vi "Main_ultra.vi"() -> ()   [LabVIEW 2020]
uses:
  <vilib>/Platform/TimedLoop/XDataNode/timing_clust.ctl
  <vilib>/Platform/TimedLoop/XDataNode/nitl_modes.ctl
  <vilib>/Platform/TimedLoop/XDataNode/wakeup.ctl
  <vilib>/Platform/TimedLoop/XDataNode/loadnilvce.vi
  <vilib>/imath/engines/lvmath2/RunTimeEngine/Managers/WorkSpace/UID Generator.vi
  <vilib>/imath/engines/lvmath2/RunTimeEngine/RunTimeType/NIMS_RunTimeType_From StrictType (excl LVString).vi
  <instcachedir>/0/NIMS_RunTimeType_From StrictType (excl LVString)_283B1B2000484AAA8744D21CE97EA49F.lvgen/NIMS_RunTimeType_From StrictType (excl LVString)_283B1B2000484AAA8744D21CE97EA49F_000.vi
  <vilib>/imath/engines/lvmath2/RunTimeEngine/LocalVariableDefStatement/MC_LocalVariableDefStatement_Display.vi
  <vilib>/imath/engines/lvmath2/RunTimeEngine/BuiltInFunctions/round/NIMS_round(DBL-S).vi
  <vilib>/imath/engines/lvmath2/RunTimeEngine/RunTimeType/NIMS_RunTimeType_Set Source Original Bool.vi
  <vilib>/imath/engines/lvmath2/RunTimeEngine/Managers/SymbolTable/Clear UID.vi
  <vilib>/imath/engines/lvmath2/RunTimeEngine/NodeEndStatement/NIMS_NodeEndStatement_Output.vi
  <instcachedir>/0/NIMS_NodeEndStatement_Output_53EC0D466D134D7ABD903AC30B43404B.lvgen/NIMS_NodeEndStatement_Output_53EC0D466D134D7ABD903AC30B43404B_001.vi
  <instcachedir>/0/NIMS_NodeEndStatement_Output_53EC0D466D134D7ABD903AC30B43404B.lvgen/NIMS_NodeEndStatement_Output_53EC0D466D134D7ABD903AC30B43404B_010.vi
  <vilib>/imath/engines/lvmath2/RunTimeEngine/ErrorHandling/NIMS_Finalize Error.vi
  Global 2.vi
  <instcachedir>/0/NIMS_NodeEndStatement_Output_53EC0D466D134D7ABD903AC30B43404B.lvgen/NIMS_NodeEndStatement_Output_53EC0D466D134D7ABD903AC30B43404B_005.vi
  <vilib>/imath/engines/lvmath2/RunTimeEngine/CommandStatement/MC_CommandStatement_break.vi
  <vilib>/imath/engines/lvmath2/RunTimeEngine/IndexReplace/NIMS M(S,S)=S.vi
  <instcachedir>/0/NIMS M(S,S)=S_FBAB070788A64735BCFA47F7F92815DB.lvgen/NIMS M(S,S)=S_FBAB070788A64735BCFA47F7F92815DB_000.vi
  <vilib>/imathl/engines/lvmath/Functions/Error Handling/Create Error.vi
  <instcachedir>/0/NIMS M(S,S)=S_FBAB070788A64735BCFA47F7F92815DB.lvgen/NIMS M(S,S)=S_FBAB070788A64735BCFA47F7F92815DB_002.vi
  <vilib>/imath/engines/lvmath2/RunTimeEngine/CommandStatement/NIMS_CommandStatement_MaskErr.vi
  <vilib>/imath/engines/lvmath2/RunTimeEngine/ArithmeticOperatorToken/NIMS_ArithmeticOperator_multmx-internal.vi
  <instcachedir>/0/NIMS_ArithmeticOperator_multmx-internal_B44B9A6937C8407A9A8862E3F2935EB3.lvgen/NIMS_ArithmeticOperator_multmx-internal_B44B9A6937C8407A9A8862E3F2935EB3_004.vi
  <vilib>/imath/engines/lvmath2/RunTimeEngine/BuiltInFunctions/length/NIMS_length(GM).vi
  <instcachedir>/0/NIMS_length(GM)_47CEC356FCE0482D9BA47DC61C99F2C7.lvgen/NIMS_length(GM)_47CEC356FCE0482D9BA47DC61C99F2C7_000.vi
  <vilib>/imath/engines/lvmath2/RunTimeEngine/RangeToken/NIMS_Range_R2 - Integer.vi
  <instcachedir>/0/NIMS_Range_R2 - Integer_FFC1A4B1B9F04947ABCB56F009996D55.lvgen/NIMS_Range_R2 - Integer_FFC1A4B1B9F04947ABCB56F009996D55_000.vi
  <vilib>/imath/engines/lvmath2/RunTimeEngine/IndexRead/NIMS M(S).vi
  <instcachedir>/0/NIMS M(S)_B826C018497E4940AE96BD27B540B6FB.lvgen/NIMS M(S)_B826C018497E4940AE96BD27B540B6FB_000.vi
  <instcachedir>/0/NIMS M(S)_B826C018497E4940AE96BD27B540B6FB.lvgen/NIMS M(S)_B826C018497E4940AE96BD27B540B6FB_005.vi
  <vilib>/imath/engines/lvmath2/RunTimeEngine/ArithmeticOperatorToken/NIMS_ArithmeticOperator_multmx(M,CV)-internal.vi
  <instcachedir>/0/NIMS_ArithmeticOperator_multmx(M,CV)-internal_19A14CC5BE0A4D31BE1E94A2E998D8C3.lvgen/NIMS_ArithmeticOperator_multmx(M,CV)-internal_19A14CC5BE0A4D31BE1E94A2E998D8C3_001.vi
  <vilib>/imath/engines/lvmath2/RunTimeEngine/IndexReplace/NIMS M($,S)=V.vi
  <instcachedir>/0/NIMS M($,S)=V_85A28EB895514E96A13A10261726EE3A.lvgen/NIMS M($,S)=V_85A28EB895514E96A13A10261726EE3A_001.vi
  <vilib>/imath/engines/lvmath2/RunTimeEngine/ErrorHandling/NIMS_Create Error From Enums.vi
  <vilib>/imath/engines/lvmath2/RunTimeEngine/RowToken/NIMS_RowToken_M_M.vi
  <instcachedir>/0/NIMS_RowToken_M_M_23B851CD98934479877138710C79658F.lvgen/NIMS_RowToken_M_M_23B851CD98934479877138710C79658F_004.vi
  <instcachedir>/0/NIMS_NodeEndStatement_Output_53EC0D466D134D7ABD903AC30B43404B.lvgen/NIMS_NodeEndStatement_Output_53EC0D466D134D7ABD903AC30B43404B_002.vi
  <vilib>/imath/engines/lvmath2/RunTimeEngine/BuiltInFunctions/size/NIMS_[I32,I32]=size(GM).vi
  <instcachedir>/0/NIMS_[I32,I32]=size(GM)_B0A6EC1255BB4C8AB801FE6F734128D9.lvgen/NIMS_[I32,I32]=size(GM)_B0A6EC1255BB4C8AB801FE6F734128D9_000.vi
  <vilib>/imath/engines/lvmath2/RunTimeEngine/BuiltInFunctions/zeros/NIMS_V=zeros(I32,I32).vi
  <vilib>/imath/engines/lvmath2/RunTimeEngine/IndexRead/NIMS M($,S).vi
  <instcachedir>/0/NIMS M($,S)_3E5749BBB62E49528D4765A77F1F6D98.lvgen/NIMS M($,S)_3E5749BBB62E49528D4765A77F1F6D98_000.vi
  <vilib>/imath/engines/lvmath2/RunTimeEngine/ArithmeticOperatorToken/NIMS_ArithmeticOperator_plus.vi
  <instcachedir>/0/NIMS_ArithmeticOperator_plus_54468E2FAC2848C4BF0D457641184E60.lvgen/NIMS_ArithmeticOperator_plus_54468E2FAC2848C4BF0D457641184E60_004.vi
  <vilib>/imath/engines/lvmath2/RunTimeEngine/RowToken/NIMS_RowToken_CV_CV.vi
  <instcachedir>/0/NIMS_RowToken_CV_CV_E2834F2F68C5494A92C49C498959A73E.lvgen/NIMS_RowToken_CV_CV_E2834F2F68C5494A92C49C498959A73E_000.vi
  <vilib>/imath/engines/lvmath2/RunTimeEngine/RowToken/NIMS_RowToken_M_CV.vi
  <instcachedir>/0/NIMS_RowToken_M_CV_79C297319A314039B767729C6880A213.lvgen/NIMS_RowToken_M_CV_79C297319A314039B767729C6880A213_000.vi
  <vilib>/imath/engines/lvmath2/RunTimeEngine/IndexRead/NIMS M(S,$).vi
  <instcachedir>/0/NIMS M(S,$)_F24F360562DE41D8BE234322A2E15C65.lvgen/NIMS M(S,$)_F24F360562DE41D8BE234322A2E15C65_000.vi
  <vilib>/imath/engines/lvmath2/RunTimeEngine/IndexReplace/NIMS M(S)=S.vi
  <instcachedir>/0/NIMS M(S)=S_033E230F5F1E47BAA81748F03F1A64B6.lvgen/NIMS M(S)=S_033E230F5F1E47BAA81748F03F1A64B6_001.vi
  <vilib>/imath/engines/lvmath2/RunTimeEngine/NodeEndStatement/NIMS_NodeEndStatement_Get Vector.vi
  <instcachedir>/0/NIMS_NodeEndStatement_Get Vector_F9EEA26507564AFBA1E30D500A99934B.lvgen/NIMS_NodeEndStatement_Get Vector_F9EEA26507564AFBA1E30D500A99934B_001.vi
  <vilib>/imath/engines/lvmath/Functions/Error Handling/MergeErrorsWrapper.vi
  <vilib>/imath/engines/lvmath2/RunTimeEngine/IndexRead/NIMS V(S).vi
  <instcachedir>/0/NIMS V(S)_0488751826AF41519A22953C041130DC.lvgen/NIMS V(S)_0488751826AF41519A22953C041130DC_000.vi
  <vilib>/imath/engines/lvmath2/RunTimeEngine/BuiltInFunctions/norm/NIMS_norm(GV,DBL).vi
  <instcachedir>/0/NIMS_norm(GV,DBL)_118B4CCB667A4D7498CD7C123070720C.lvgen/NIMS_norm(GV,DBL)_118B4CCB667A4D7498CD7C123070720C_000.vi
  <vilib>/imath/engines/lvmath2/RunTimeEngine/BuiltInFunctions/cos/NIMS_cos(C).vi
  <instcachedir>/0/NIMS_cos(C)_9DC0D0878EF24EB8B280F2BED1FF8FCD.lvgen/NIMS_cos(C)_9DC0D0878EF24EB8B280F2BED1FF8FCD_001.vi
  <vilib>/imath/engines/lvmath2/RunTimeEngine/BuiltInFunctions/acos/NIMS_acos(C).vi
  <instcachedir>/0/NIMS_acos(C)_5BB0E87CCFB0408A9DC8B350AC83525E.lvgen/NIMS_acos(C)_5BB0E87CCFB0408A9DC8B350AC83525E_001.vi
  <instcachedir>/0/NIMS_RunTimeType_From StrictType (excl LVString)_283B1B2000484AAA8744D21CE97EA49F.lvgen/NIMS_RunTimeType_From StrictType (excl LVString)_283B1B2000484AAA8744D21CE97EA49F_009.vi
  <vilib>/imath/engines/lvmath2/RunTimeEngine/BuiltInFunctions/abs/NIMS_abs(signed).vi
  <instcachedir>/0/NIMS_abs(signed)_C4FCB8E6058B49B797C7C8D53CA5F6EC.lvgen/NIMS_abs(signed)_C4FCB8E6058B49B797C7C8D53CA5F6EC_002.vi
  <instcachedir>/0/NIMS_NodeEndStatement_Output_53EC0D466D134D7ABD903AC30B43404B.lvgen/NIMS_NodeEndStatement_Output_53EC0D466D134D7ABD903AC30B43404B_009.vi
  <vilib>/platform/TimedLoop/XDataNode/XDataNode.xnode
  <vilib>/Platform/TimedLoop/XDataNode/XDNodeRunTimeDep.lvlib
  <vilib>/imath/engines/lvmath2/RunTimeEngine/Managers/SymbolTable/NIMS_WorkSpace.lvlib
panel:
  out "Temperature":dbl=43.13496907791888
  out "VoltageSaturating":bool
  out "Power":bool
  in  "Power On/Off":bool
  in  "BMagnitude [T]":dbl=0.02
  out "RotationPerSecond[Hz]":dbl=-94.24777499999999
  in  "RotationsPerSecond [Hz]":dbl=-20.0
  out "AngleX":cluster{dbl, dbl}(graph)
  in  "Max Orientation\n change rate [rad/s]":dbl=30.0
  in  "Force Vertical":bool
  in  "Scalar":dbl=0.004
  out "F":dbl=-596.1678650885794
  in  "Reset Integral":bool
  in  "Kp":dbl=40.0
  in  "Ki":dbl=0.001
  in  "Kd":dbl
  out "XY View":T1(graph)=[{"XCircleBot"=[0.03623369648886077, 0.03598886161264151, 0.035314301100597044, 0.034375170892196175, 0.03340140281576648, 0.0326314092577669, 0.03225371149565987, 0.032360783114279174, 0.03292640924713354, 0.03381210488999921, 0.034801020859787216, 0.03565103603744329, 0.0361540370621615], "YCircleBot"=[0.0012174224381933385, 0.0021762735154017446, 0.002900364407809132, 0.0032124124114014476, 0.0030360172918447023, 0.002414366726401252, 0.001499662454313073, 0.0005158559828140988, -0.00029618255242251797, -0.0007376377971368554, -0.0007004261111329384, -0.00019365821294744547, 0.0006585914417954867]}, {"XCircleBot"=[0.0, -0.00199, -0.004019999999999999, -0.0061200000000000004, -0.00816, -0.01026, -0.01234, -0.01435, -0.01622, -0.01804, -0.019920000000000004, -0.02168, -0.02325, -0.02478, -0.02623, -0.02775, -0.02913, -0.030440000000000002, -0.03164, -0.032729999999999995, -0.0337, -0.03456, -0.03524, -0.035840000000000004, -0.03629, -0.03668, -0.03701, -0.03726, -0.037469999999999996, -0.037590000000000005, -0.037630000000000004, -0.03762, -0.03754, -0.037450000000000004, -0.03697, -0.03612, -0.03502, -0.03358, -0.03181, -0.029840000000000002, -0.027800000000000002, -0.0257, -0.023629999999999998, -0.02158, -0.01957, -0.01754, -0.01551, -0.01343, -0.01131, -0.00925, -0.00714, -0.00525, -0.0035499999999999998, -0.00213, -0.0010500000000000002, -0.00041, -3e-05, 0.00047, 0.00132, 0.00252, 0.00405, 0.0057599999999999995, 0.00772, 0.00973, 0.01173, 0.013960000000000002, 0.0162, 0.01825, 0.02047, 0.02266, 0.02475, 0.026760000000000003, 0.028820000000000002, 0.03086, 0.03277, 0.03442, 0.0357, 0.0366, 0.037200000000000004, 0.037520000000000005, 0.03764, 0.037649999999999996, 0.037590000000000005, 0.037520000000000005, 0.037469999999999996, 0.03746, 0.037469999999999996, 0.03749, 0.0375, 0.03751, 0.03751, 0.03751, 0.03751, 0.03751, 0.0375, 0.0375, 0.0375, 0.0375, 0.0375, 0.0375, 0.0375, 0.0375, 0.0375, 0.0375, 0.0375, 0.0375, 0.0375, 0.0375, 0.0375, 0.0375, 0.0375, 0.0375, 0.0375, 0.0375, 0.0375, 0.0375, 0.0375, 0.03751, 0.03751, 0.0375, 0.03748, 0.037469999999999996, 0.037469999999999996, 0.03746, 0.03746, 0.037469999999999996, 0.03749, 0.03753, 0.03758, 0.037630000000000004, 0.03764, 0.0375, 0.03712, 0.03649, 0.0356, 0.034350000000000006, 0.03275, 0.0308, 0.02878, 0.02666, 0.02456, 0.02236, 0.02014, 0.01796, 0.01591, 0.01368, 0.01167, 0.009519999999999999, 0.00723, 0.00479, 0.0027300000000000002, 0.0005600000000000001, 0.0], "YCircleBot"=[-0.0375, -0.03775, -0.03756, -0.03716, -0.03663, -0.03598, -0.035250000000000004, -0.03448, -0.0337, -0.03286, -0.03188, -0.03074, -0.02947, -0.028059999999999998, -0.02664, -0.025050000000000003, -0.0235, -0.02189, -0.020239999999999998, -0.01853, -0.01672, -0.01477, -0.01286, -0.01078, -0.00881, -0.0067800000000000004, -0.004730000000000001, -0.00269, -0.00048, 0.00161, 0.00372, 0.0057599999999999995, 0.00785, 0.009869999999999999, 0.01182, 0.01365, 0.0154, 0.01682, 0.01777, 0.0183, 0.018600000000000002, 0.01875, 0.01881, 0.01881, 0.01877, 0.01871, 0.0187, 0.01878, 0.01886, 0.018760000000000002, 0.01833, 0.01753, 0.016370000000000003, 0.01494, 0.01318, 0.01114, 0.00903, 0.0069500000000000004, 0.00512, 0.0034700000000000004, 0.0020099999999999996, 0.00092, 0.0003, 8e-05, 1e-05, -2e-05, -3e-05, -3e-05, -2e-05, -1e-05, 0.0, 0.0, 0.0, 0.0, 0.0, 0.0, 0.0, 0.0, 0.0, 0.0, 0.0, 0.0, 0.0, 0.0, 1e-05, 1e-05, 2e-05, 1e-05, 0.0, -2e-05, -5e-05, -8.999999999999999e-05, -0.00016, -0.00025, -0.00039000000000000005, -0.00063, -0.0011899999999999999, -0.00279, -0.00452, -0.00628, -0.008150000000000001, -0.01018, -0.01219, -0.01428, -0.016329999999999997, -0.01837, -0.020489999999999998, -0.022600000000000002, -0.02475, -0.02677, -0.02884, -0.03083, -0.03264, -0.03432, -0.03574, -0.03672, -0.0373, -0.03749, -0.0375, -0.0375, -0.0375, -0.0375, -0.0375, -0.0375, -0.0375, -0.0375, -0.0375, -0.0375, -0.0375, -0.0375, -0.0375, -0.0375, -0.0375, -0.0375, -0.0375, -0.0375, -0.0375, -0.0375, -0.0375, -0.0375, -0.0375, -0.0375, -0.0375, -0.0375, -0.0375, -0.0375, -0.0375, -0.0375, -0.0375, -0.0375, -0.0375, -0.0375, -0.0375]}, {"XCircleBot"=[0.02876, 0.028515165123780748, 0.02784060461173628, 0.02690147440333541, 0.025927706326905716, 0.025157712768906135, 0.024780015006799112, 0.02488708662541841, 0.02545271275827278, 0.026338408401138443, 0.027327324370926456, 0.028177339548582522, 0.028680340573300735], "YCircleBot"=[0.0, 0.000958851077208406, 0.0016829419696157931, 0.001994989973208109, 0.0018185948536513636, 0.0011969442882079132, 0.0002822400161197344, -0.0007015664553792397, -0.0015136049906158565, -0.001955060235330194, -0.001917848549326277, -0.001411080651140784, -0.0005588309963978518]}, {"XCircleBot"=[0.034233696488860765, 0.035873148282011894], "YCircleBot"=[0.0012174224381933385, 0.0004059623274943767]}]
  out "XZ View":T1(graph)=[{"XCircleBot"=[0.03623369648886077, 0.03598886161264151, 0.035314301100597044, 0.034375170892196175, 0.03340140281576648, 0.0326314092577669, 0.03225371149565987, 0.032360783114279174, 0.03292640924713354, 0.03381210488999921, 0.034801020859787216, 0.03565103603744329, 0.0361540370621615], "YCircleBot"=[-0.07416133745930864, -0.07320248638210024, -0.07247839548969284, -0.07216634748610053, -0.07234274260565728, -0.07296439317110073, -0.0738790974431889, -0.07486290391468788, -0.0756749424499245, -0.07611639769463883, -0.07607918600863492, -0.07557241811044943, -0.07472016845570649]}, {"XCircleBot"=[0.0, -0.00199, -0.004019999999999999, -0.0061200000000000004, -0.00816, -0.01026, -0.01234, -0.01435, -0.01622, -0.01804, -0.019920000000000004, -0.02168, -0.02325, -0.02478, -0.02623, -0.02775, -0.02913, -0.030440000000000002, -0.03164, -0.032729999999999995, -0.0337, -0.03456, -0.03524, -0.035840000000000004, -0.03629, -0.03668, -0.03701, -0.03726, -0.037469999999999996, -0.037590000000000005, -0.037630000000000004, -0.03762, -0.03754, -0.037450000000000004, -0.03697, -0.03612, -0.03502, -0.03358, -0.03181, -0.029840000000000002, -0.027800000000000002, -0.0257, -0.023629999999999998, -0.02158, -0.01957, -0.01754, -0.01551, -0.01343, -0.01131, -0.00925, -0.00714, -0.00525, -0.0035499999999999998, -0.00213, -0.0010500000000000002, -0.00041, -3e-05, 0.00047, 0.00132, 0.00252, 0.00405, 0.0057599999999999995, 0.00772, 0.00973, 0.01173, 0.013960000000000002, 0.0162, 0.01825, 0.02047, 0.02266, 0.02475, 0.026760000000000003, 0.028820000000000002, 0.03086, 0.03277, 0.03442, 0.0357, 0.0366, 0.037200000000000004, 0.037520000000000005, 0.03764, 0.037649999999999996, 0.037590000000000005, 0.037520000000000005, 0.037469999999999996, 0.03746, 0.037469999999999996, 0.03749, 0.0375, 0.03751, 0.03751, 0.03751, 0.03751, 0.03751, 0.0375, 0.0375, 0.0375, 0.0375, 0.0375, 0.0375, 0.0375, 0.0375, 0.0375, 0.0375, 0.0375, 0.0375, 0.0375, 0.0375, 0.0375, 0.0375, 0.0375, 0.0375, 0.0375, 0.0375, 0.0375, 0.0375, 0.0375, 0.03751, 0.03751, 0.0375, 0.03748, 0.037469999999999996, 0.037469999999999996, 0.03746, 0.03746, 0.037469999999999996, 0.03749, 0.03753, 0.03758, 0.037630000000000004, 0.03764, 0.0375, 0.03712, 0.03649, 0.0356, 0.034350000000000006, 0.03275, 0.0308, 0.02878, 0.02666, 0.02456, 0.02236, 0.02014, 0.01796, 0.01591, 0.01368, 0.01167, 0.009519999999999999, 0.00723, 0.00479, 0.0027300000000000002, 0.0005600000000000001, 0.0], "YCircleBot"=[0.0, 0.0, 0.0, 0.0, 0.0, 0.0, 0.0, 0.0, 0.0, 0.0, 0.0, 0.0, 0.0, 0.0, 0.0, 0.0, 0.0, 0.0, 0.0, 0.0, 0.0, 0.0, 0.0, 0.0, 0.0, 0.0, 0.0, 0.0, 0.0, 0.0, 0.0, 0.0, 0.0, 0.0, 0.0, 0.0, 0.0, 0.0, 0.0, 0.0, 0.0, 0.0, 0.0, 0.0, 0.0, 0.0, 0.0, 0.0, 0.0, 0.0, 0.0, 0.0, 0.0, 0.0, 0.0, 0.0, 0.0, 0.0, 0.0, 0.0, 0.0, 0.0, 0.0, 0.0, 0.0, 0.0, 1e-05, 1e-05, 1e-05, 1e-05, -1e-05, -4e-05, 0.00017, 0.00063, 0.00143, 0.0027, 0.00435, 0.00619, 0.00816, 0.01016, 0.012230000000000001, 0.01425, 0.01629, 0.0183, 0.02036, 0.0224, 0.02442, 0.02655, 0.028800000000000003, 0.03081, 0.032979999999999995, 0.03522, 0.03744, 0.039549999999999995, 0.0417, 0.04382, 0.045770000000000005, 0.047, 0.048049999999999995, 0.04915, 0.049890000000000004, 0.05004, 0.04999, 0.04997, 0.04998, 0.04999, 0.05001, 0.05002, 0.05002, 0.05001, 0.04995, 0.049479999999999996, 0.04846, 0.047200000000000006, 0.045700000000000005, 0.043930000000000004, 0.042, 0.039939999999999996, 0.037880000000000004, 0.03587, 0.03356, 0.03125, 0.02913, 0.026949999999999998, 0.02477, 0.02266, 0.02036, 0.01833, 0.016100000000000003, 0.014060000000000001, 0.012029999999999999, 0.01, 0.00795, 0.006030000000000001, 0.00421, 0.0025499999999999997, 0.00132, 0.00055, 0.00017999999999999998, 3e-05, -2e-05, -2e-05, 1e-05, 4e-05, 7.000000000000001e-05, 8.999999999999999e-05, 0.0001, 0.00011, 0.0001, 8e-05, 5e-05, 1e-05, 0.0]}, {"XCircleBot"=[0.02876, 0.028515165123780748, 0.02784060461173628, 0.02690147440333541, 0.025927706326905716, 0.025157712768906135, 0.024780015006799112, 0.02488708662541841, 0.02545271275827278, 0.026338408401138443, 0.027327324370926456, 0.028177339548582522, 0.028680340573300735], "YCircleBot"=[-4e-05, 0.000918851077208406, 0.001642941969615793, 0.001954989973208109, 0.0017785948536513635, 0.001156944288207913, 0.0002422400161197344, -0.0007415664553792397, -0.0015536049906158566, -0.001995060235330194, -0.001957848549326277, -0.001451080651140784, -0.0005988309963978518]}, {"XCircleBot"=[0.034233696488860765, 0.035873148282011894], "YCircleBot"=[-0.07416133745930864, -0.024194811361262974]}]
  in  "Ahead":dbl=1.0 format="%#_13g"
  out "Error":dbl(graph)=0.07450711995076267
  out "error":cdb=0.07450711995076267+0.0i
  in  "Radio Buttons":enum32{"Stadium", "Circle"}(radio)
  in  "Zscale":dbl=0.95
  in  "YScale":dbl=0.9
  in  "XScale":dbl=0.95
  in  "Zoffset":dbl=-0.073
  in  "Yoffset":dbl=-0.076
  in  "Xoffset":dbl=0.07
  in  "Traj_Rotate":bool
  in  "stop":bool
  out "Loop Duration [ms]":u32
  in  "Settings 4":T2={"Objects"=1, "Threshold"=95, "Reject Border"=FALSE, "Fill Holes"=FALSE, "Min Object Size"=TRUE, "Min Size"=25, "Max Object Size"=TRUE, "Max Size"=25000, "Show Search Area"=TRUE, "Show Center"=TRUE, "Show Bounding Box"=TRUE} {"Objects" items=["Bright Objects", "Dark Objects"]; "Threshold" min=1 max=999999999 step=1; "Max Size" min=1 max=999999999 step=1; "Min Size" min=1 max=999999999 step=1}
  out "Image 4":T3(plugin-control)
  in  "Settings 3":T2={"Objects"=1, "Threshold"=1, "Reject Border"=FALSE, "Fill Holes"=FALSE, "Min Object Size"=TRUE, "Min Size"=25, "Max Object Size"=TRUE, "Max Size"=25000, "Show Search Area"=FALSE, "Show Center"=TRUE, "Show Bounding Box"=TRUE} {"Objects" items=["Bright Objects", "Dark Objects"]; "Threshold" min=1 max=999999999 step=1; "Max Size" min=1 max=999999999 step=1; "Min Size" min=1 max=999999999 step=1}
  out "Image 3":T3(plugin-control)
  in  "Vision compensation":bool=TRUE
  out "Vision compensation active":bool=TRUE
  out "coordinates":cluster{dbl, dbl, dbl}(graph)={0.0027, -0.0171, 0.0805}
  out "camera rate":u32=11
  out "X":dbl=0.0027
  out "Y":dbl=-0.0171
  out "Z":dbl=0.0805
  out "Error_detection":bool
  out "Detection_Error":cdb
  in  "Search Rect (entire image)":T4={"Left"=224, "Top"=459, "Right"=496, "Bottom"=249, "Rotation"=0.0} {"Rotation" format="%.2f"; "Left" scale=0.0..1024.0; "Right" scale=0.0..1024.0}
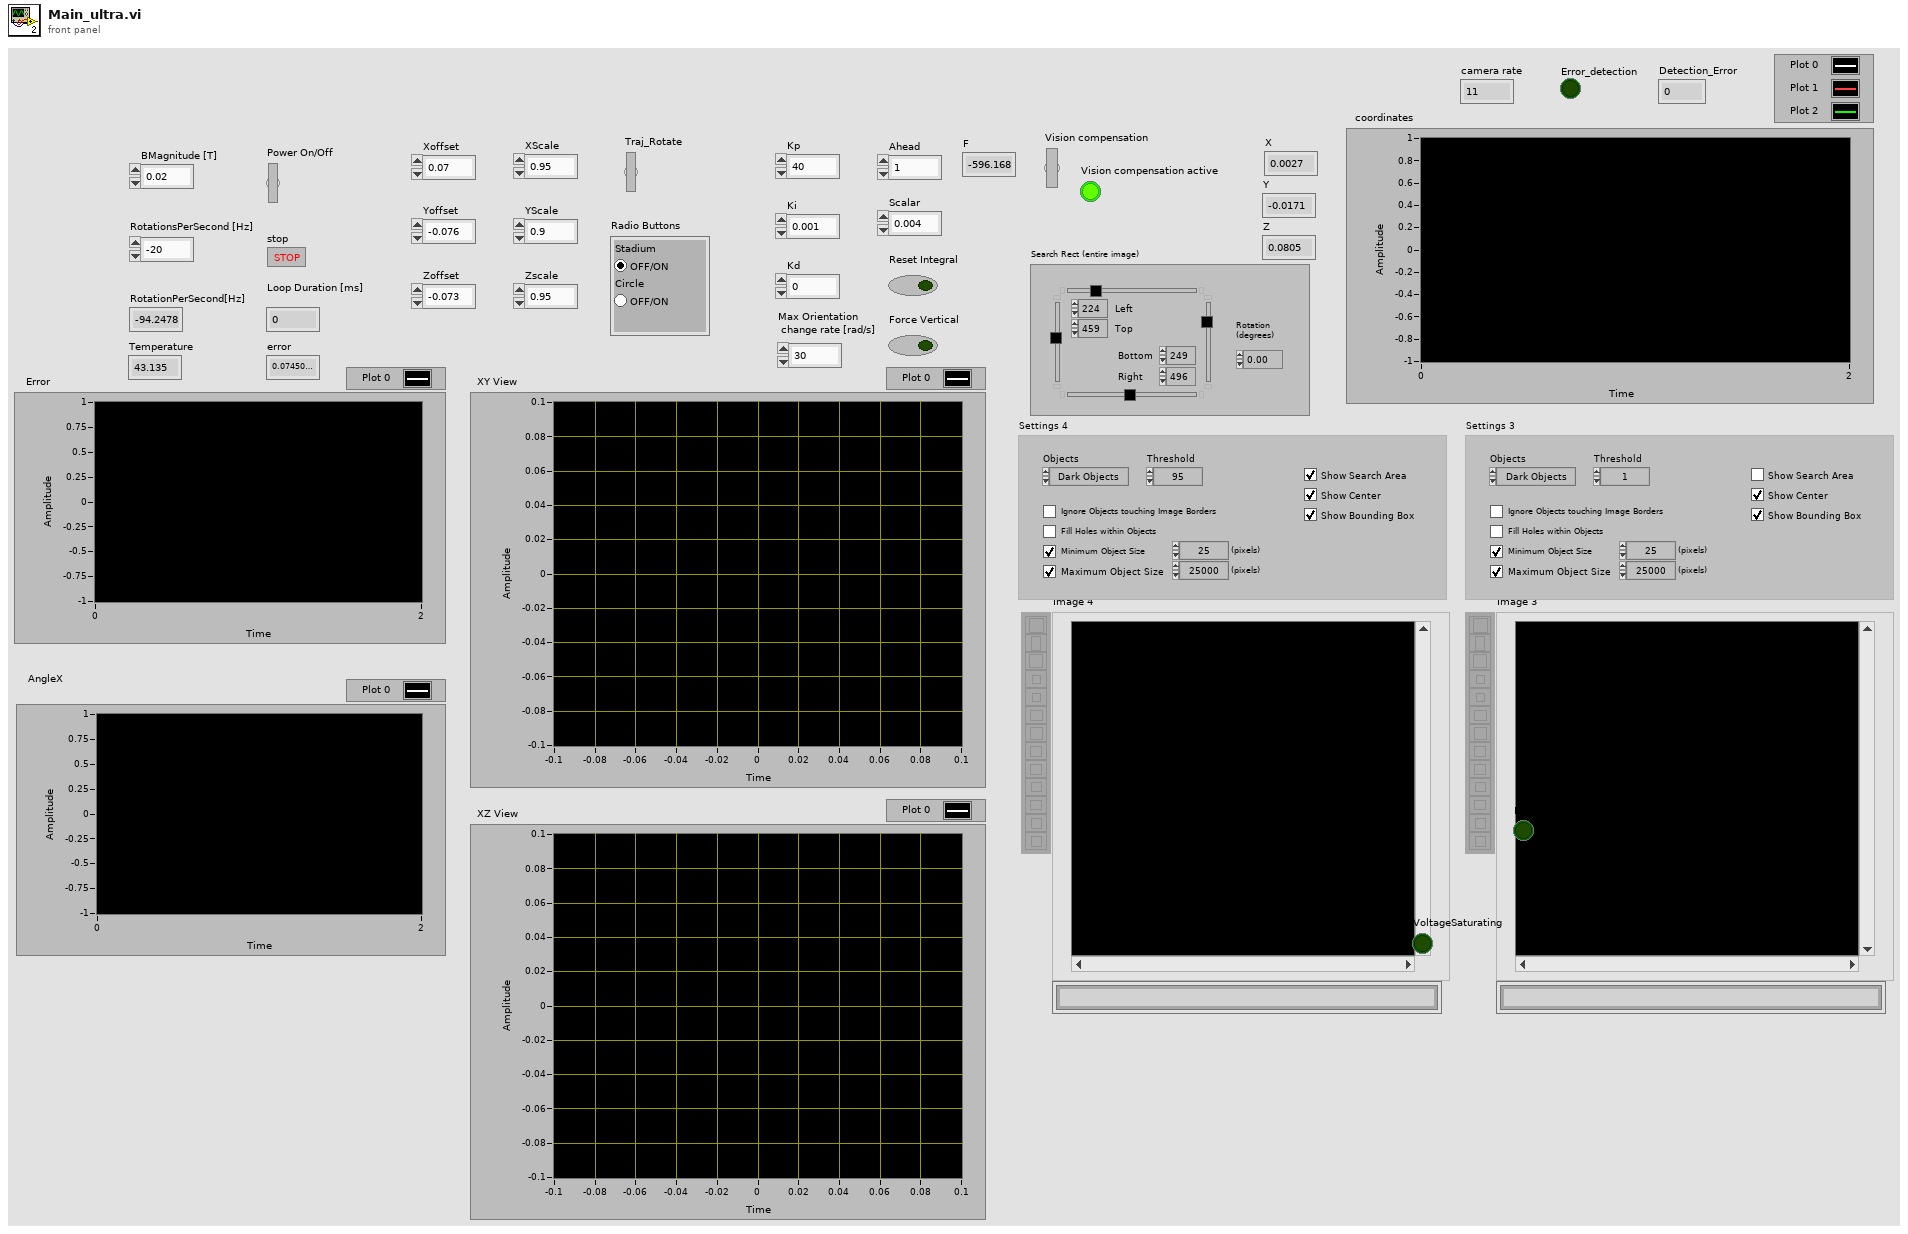
[diagram p1: front panel]
types:
  T1 = cluster{"XCircleBot":dbl[], "YCircleBot":dbl[]}[]
  T2 = cluster{"Objects":u16, "Threshold":i32, "Reject Border":bool, "Fill Holes":bool, "Min Object Size":bool, "Min Size":i32, "Max Object Size":bool, "Max Size":i32, "Show Search Area":bool, "Show Center":bool, "Show Bounding Box":bool}
  T3 = typedef "IMAQ Image.ctl" = refnum<image>
  T4 = typedef "IMAQ Rectangle" = cluster{"Left":i32, "Top":i32, "Right":i32, "Bottom":i32, "Rotation":dbl}
  T5 = typedef "XDNodeRunTimeDep.lvlib/timing_clust.ctl" = cluster{"Expected End [f-1]":u64, "Actual End [f-1]":u64, "Finished Late? [f-1]":bool, "Expected End [i-1]":u64, "Actual End [i-1]":u64, "Finished Late? [i-1]":bool, "Expected Start [i]":u64, "Actual Start [i]":u64, "Expected Start [f]":u64, "Actual Start [f]":u64, "Source Name":string, "Structure Name":string, "Period":i64, "Deadline":i64, "Offset":i64, "Start":i64, "Priority":i32, "Timeout":i32, "Mode":T6, "Wakeup Reason":T7, "Error":errorcluster, "Source Type":string, "Secondary Source Type":string, "Global End Time":u64, "Global Start Time":u64, "Frame Duration":u64, "Iteration Duration":u64, "Assigned CPU":i32, "I/O Scan Engine Mode":u32}
  T6 = typedef "XDNodeRunTimeDep.lvlib/nitl_modes.ctl" = enum32{"No Change", "Process missed periods, maintain original phase", "Discard missed periods, maintain original phase", "Process missed periods, ignore original phase", "Discard missed periods, ignore original phase"}
  T7 = typedef "XDNodeRunTimeDep.lvlib/wakeup.ctl" = enum32{"Normal", "Aborted", "Asynchronous wakeup", "Timing source error", "Timed loop error", "Timeout"}
  T8 = cluster{"XCircleClosestOut":dbl[], "ZCircleClosestOut":dbl[]}
  T9 = cluster{"XCircleBotOut":dbl[], "ZCircleBotOut":dbl[]}
  T10 = cluster{"XCircleClosestOut":dbl[], "YCircleClosestOut":dbl[]}
  T11 = cluster{"XCircleBotOut":dbl[], "YCircleBotOut":dbl[]}
  T12 = cluster{cluster{"XCircleBotOut":dbl[], "YCircleBotOut":dbl[]}, cluster{"XHD":dbl[], "YHD":dbl[]}, cluster{"XCircleClosestOut":dbl[], "YCircleClosestOut":dbl[]}, cluster{"XPlot":dbl[], "YPlot":dbl[]}}
  T13 = cluster{cluster{"XCircleBotOut":dbl[], "ZCircleBotOut":dbl[]}, cluster{"XHD":dbl[], "ZHD":dbl[]}, cluster{"XCircleClosestOut":dbl[], "ZCircleClosestOut":dbl[]}, cluster{"XPlot":dbl[], "ZPlot":dbl[]}}
  T14 = cluster{"Object Center":cluster{"X":sgl, "Y":sgl}, "Bounding Box":cluster{"X Left":i32, "Y Top":i32, "X Right":i32, "Y Bottom":i32}, "Area":sgl, "Orientation":sgl, "Aspect Ratio":sgl, "Nb Holes":i32}[]
  T15 = cluster{"Objects[0]":cluster{"Object Center":cluster{"X":sgl, "Y":sgl}, "Bounding Box":cluster{"X Left":i32, "Y Top":i32, "X Right":i32, "Y Bottom":i32}, "Area":sgl, "Orientation":sgl, "Aspect Ratio":sgl, "Nb Holes":i32}, "Objects[1]":cluster{"Object Center":cluster{"X":sgl, "Y":sgl}, "Bounding Box":cluster{"X Left":i32, "Y Top":i32, "X Right":i32, "Y Bottom":i32}, "Area":sgl, "Orientation":sgl, "Aspect Ratio":sgl, "Nb Holes":i32}, "Objects[2]":cluster{"Object Center":cluster{"X":sgl, "Y":sgl}, "Bounding Box":cluster{"X Left":i32, "Y Top":i32, "X Right":i32, "Y Bottom":i32}, "Area":sgl, "Orientation":sgl, "Aspect Ratio":sgl, "Nb Holes":i32}, "Objects[3]":cluster{"Object Center":cluster{"X":sgl, "Y":sgl}, "Bounding Box":cluster{"X Left":i32, "Y Top":i32, "X Right":i32, "Y Bottom":i32}, "Area":sgl, "Orientation":sgl, "Aspect Ratio":sgl, "Nb Holes":i32}, "Objects[4]":cluster{"Object Center":cluster{"X":sgl, "Y":sgl}, "Bounding Box":cluster{"X Left":i32, "Y Top":i32, "X Right":i32, "Y Bottom":i32}, "Area":sgl, "Orientation":sgl, "Aspect Ratio":sgl, "Nb Holes":i32}, "Objects[5]":cluster{"Object Center":cluster{"X":sgl, "Y":sgl}, "Bounding Box":cluster{"X Left":i32, "Y Top":i32, "X Right":i32, "Y Bottom":i32}, "Area":sgl, "Orientation":sgl, "Aspect Ratio":sgl, "Nb Holes":i32}, "Objects[6]":cluster{"Object Center":cluster{"X":sgl, "Y":sgl}, "Bounding Box":cluster{"X Left":i32, "Y Top":i32, "X Right":i32, "Y Bottom":i32}, "Area":sgl, "Orientation":sgl, "Aspect Ratio":sgl, "Nb Holes":i32}, "Objects[7]":cluster{"Object Center":cluster{"X":sgl, "Y":sgl}, "Bounding Box":cluster{"X Left":i32, "Y Top":i32, "X Right":i32, "Y Bottom":i32}, "Area":sgl, "Orientation":sgl, "Aspect Ratio":sgl, "Nb Holes":i32}, "Objects[8]":cluster{"Object Center":cluster{"X":sgl, "Y":sgl}, "Bounding Box":cluster{"X Left":i32, "Y Top":i32, "X Right":i32, "Y Bottom":i32}, "Area":sgl, "Orientation":sgl, "Aspect Ratio":sgl, "Nb Holes":i32}}
  T16 = cluster{"Object Center":cluster{"X":sgl, "Y":sgl}, "Bounding Box":cluster{"X Left":i32, "Y Top":i32, "X Right":i32, "Y Bottom":i32}, "Area":sgl, "Orientation":sgl, "Aspect Ratio":sgl, "Nb Holes":i32}
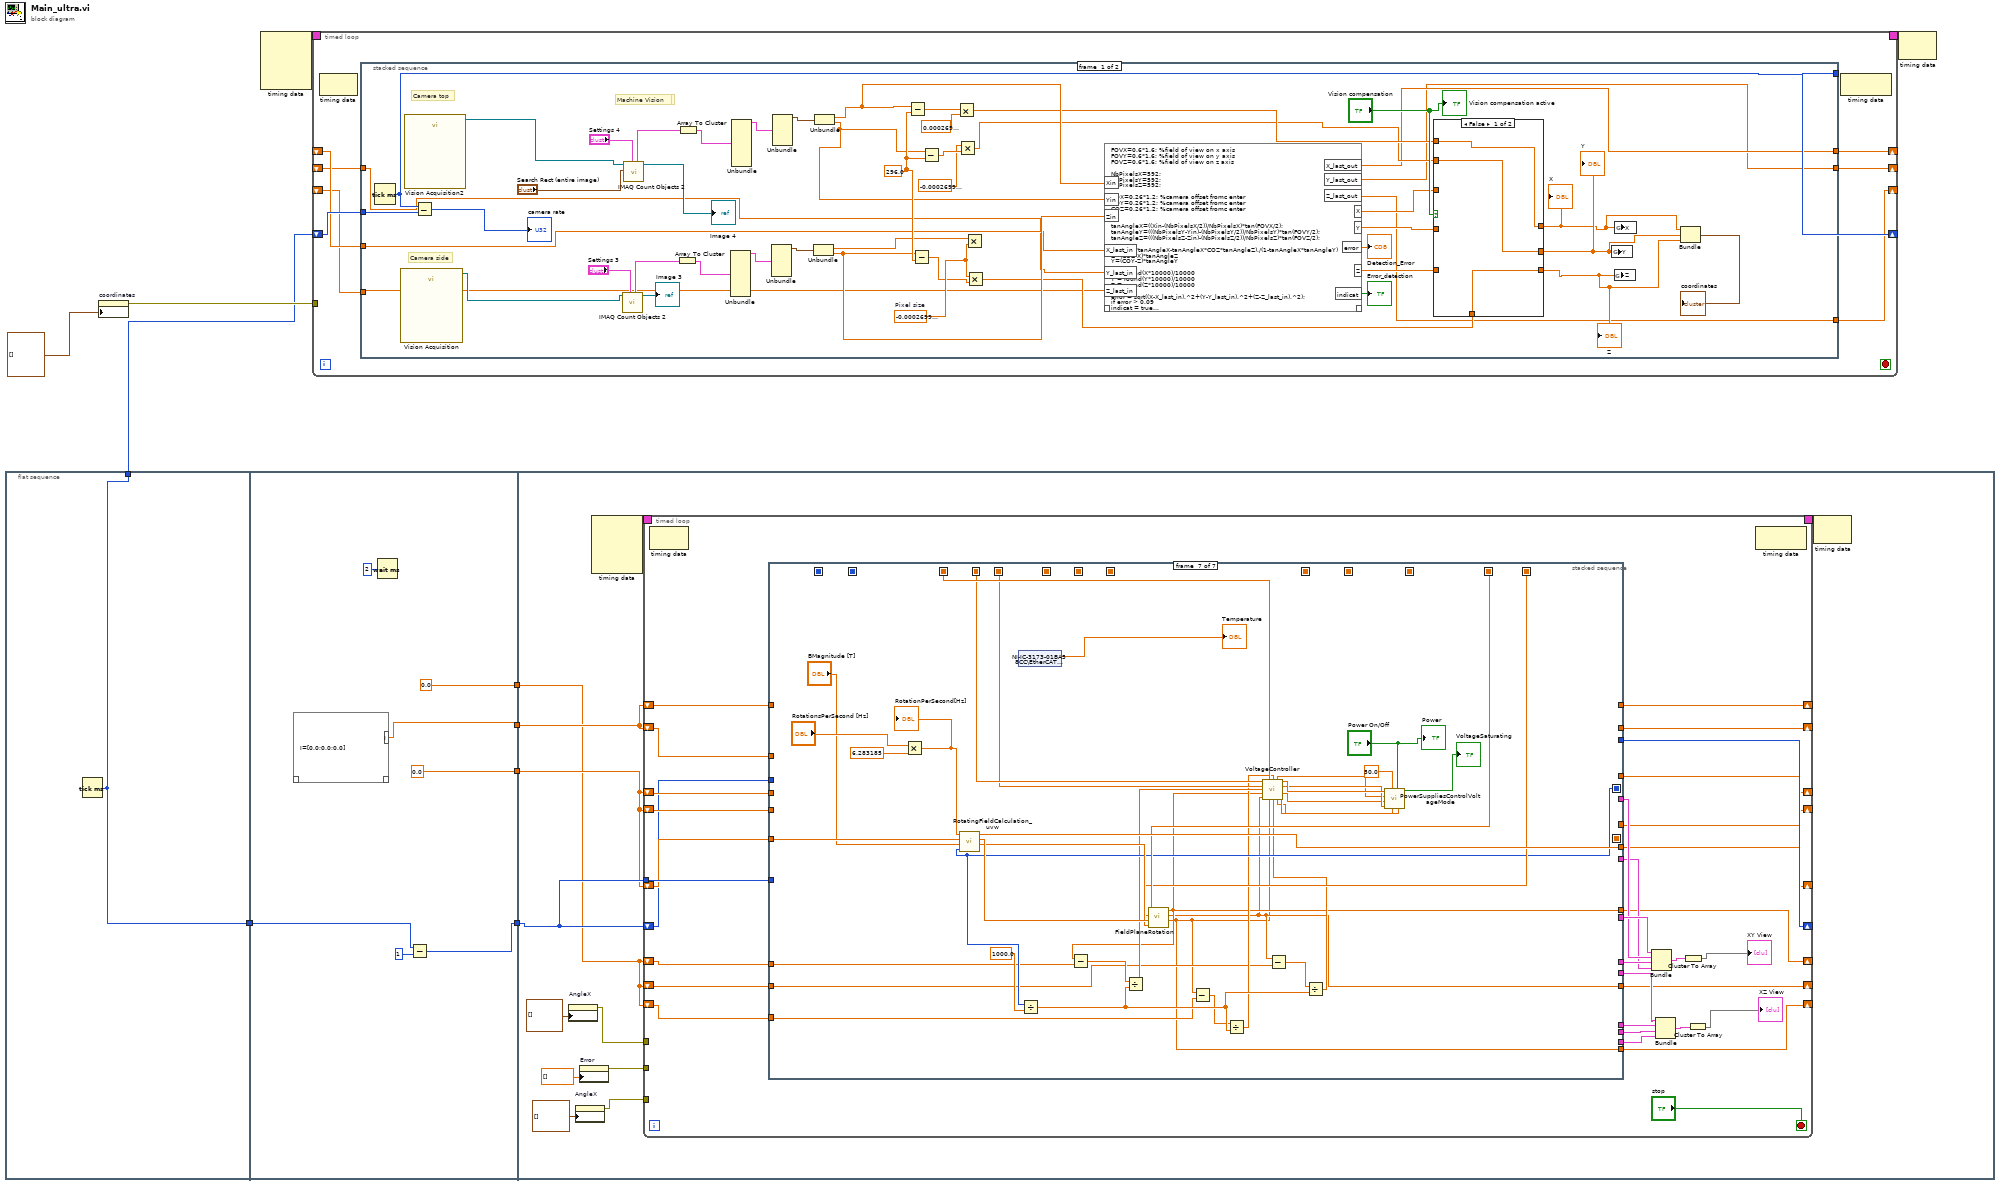
[diagram p0: block diagram]
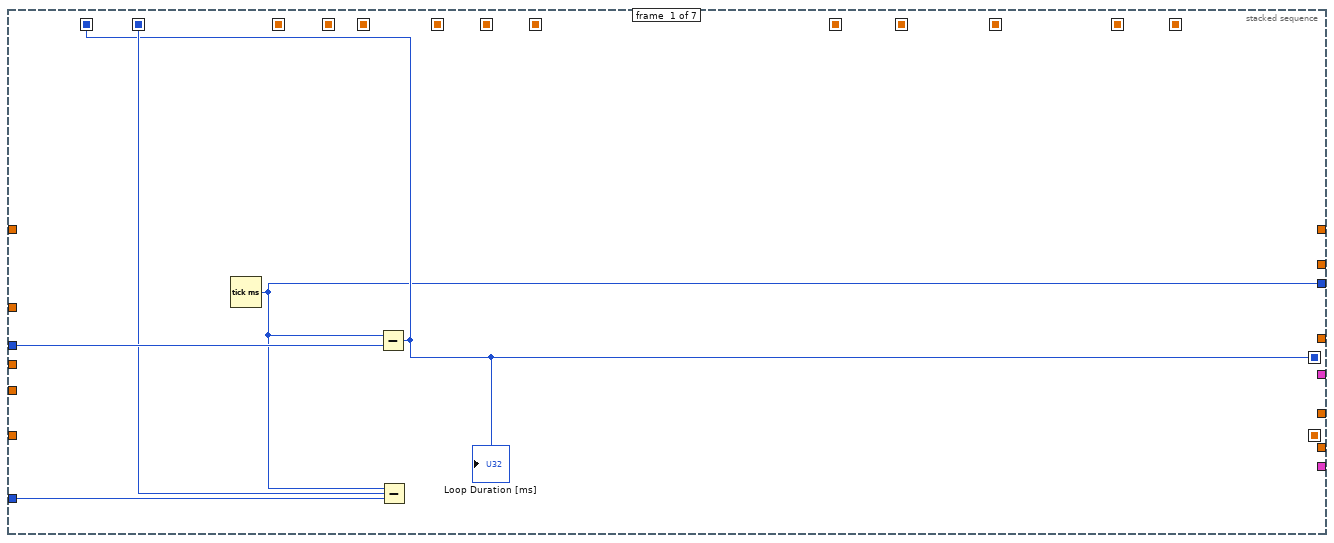
[diagram p2: hidden frame]
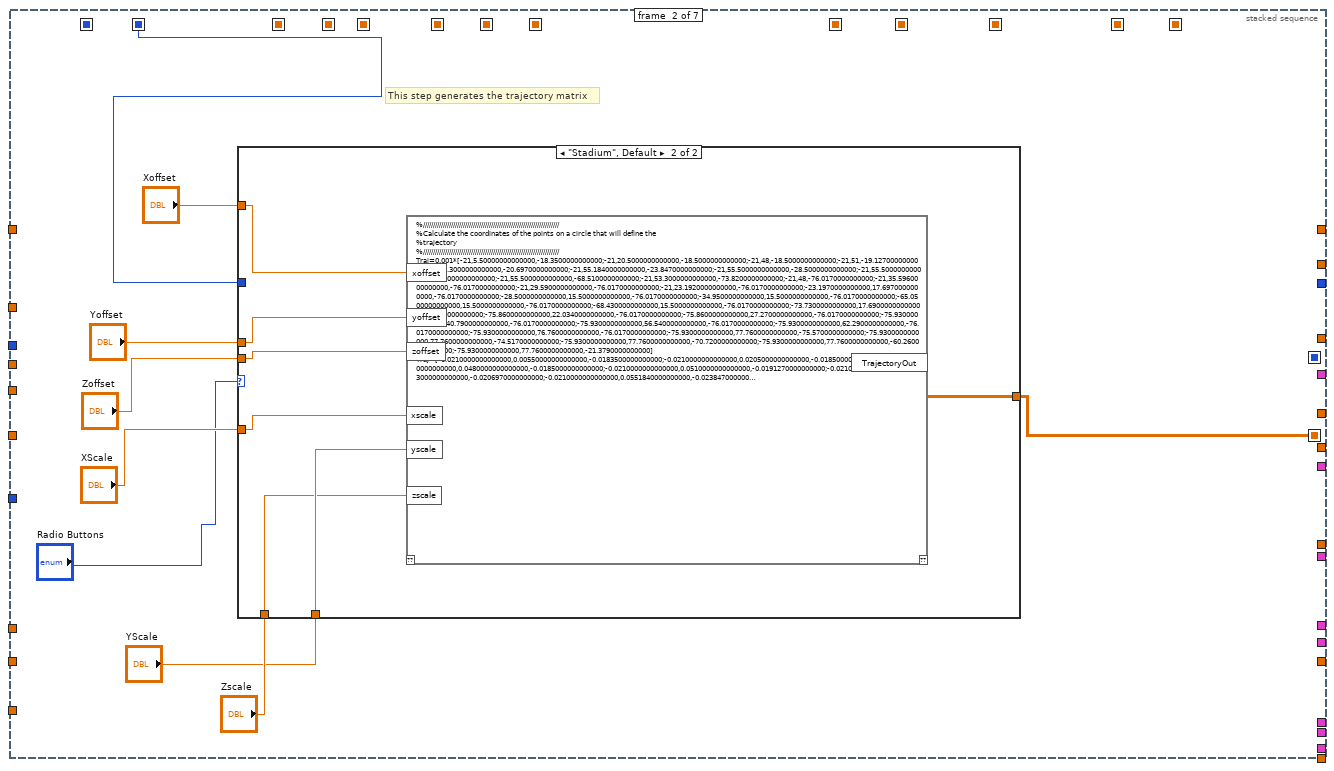
[diagram p3: hidden frame]
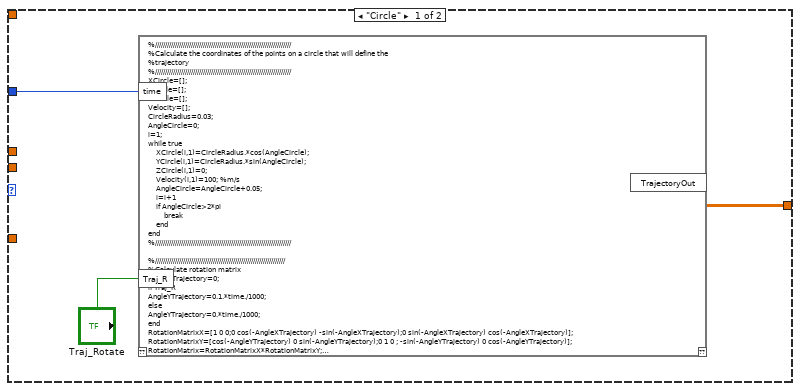
[diagram p4: hidden frame]
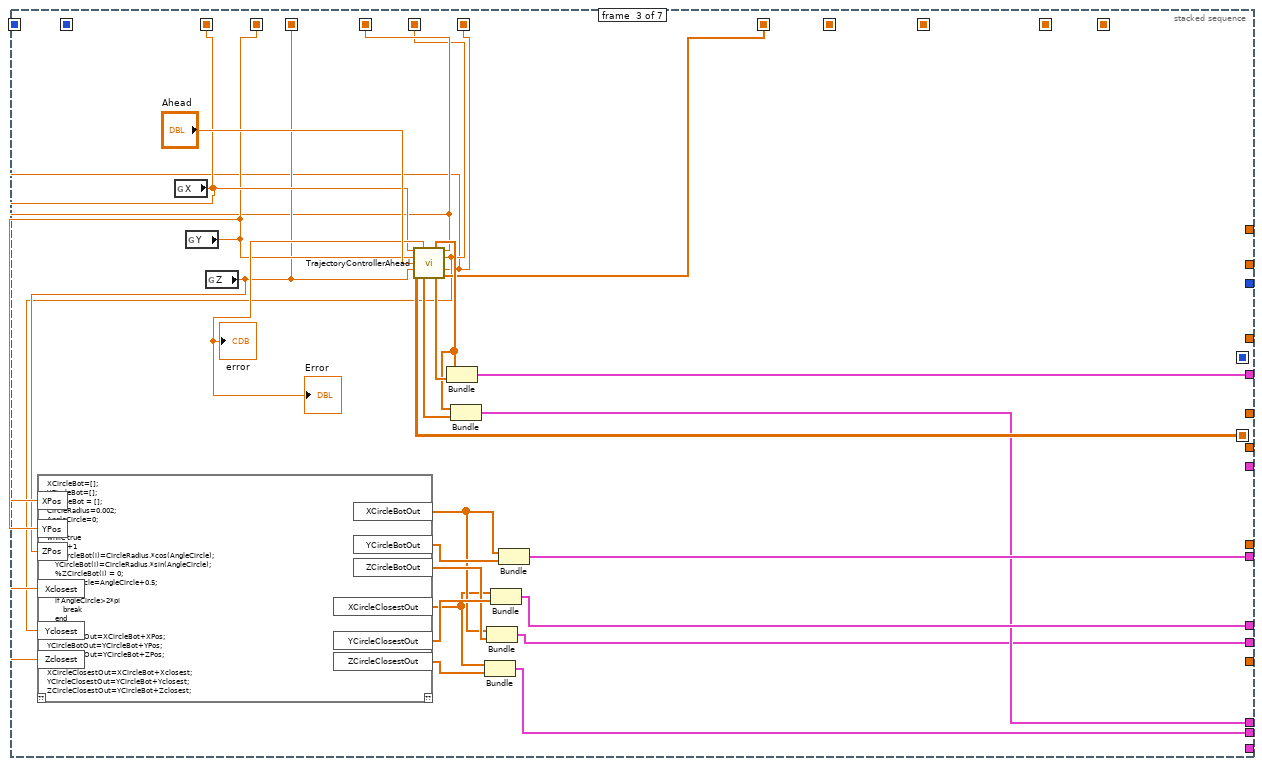
[diagram p5: hidden frame]
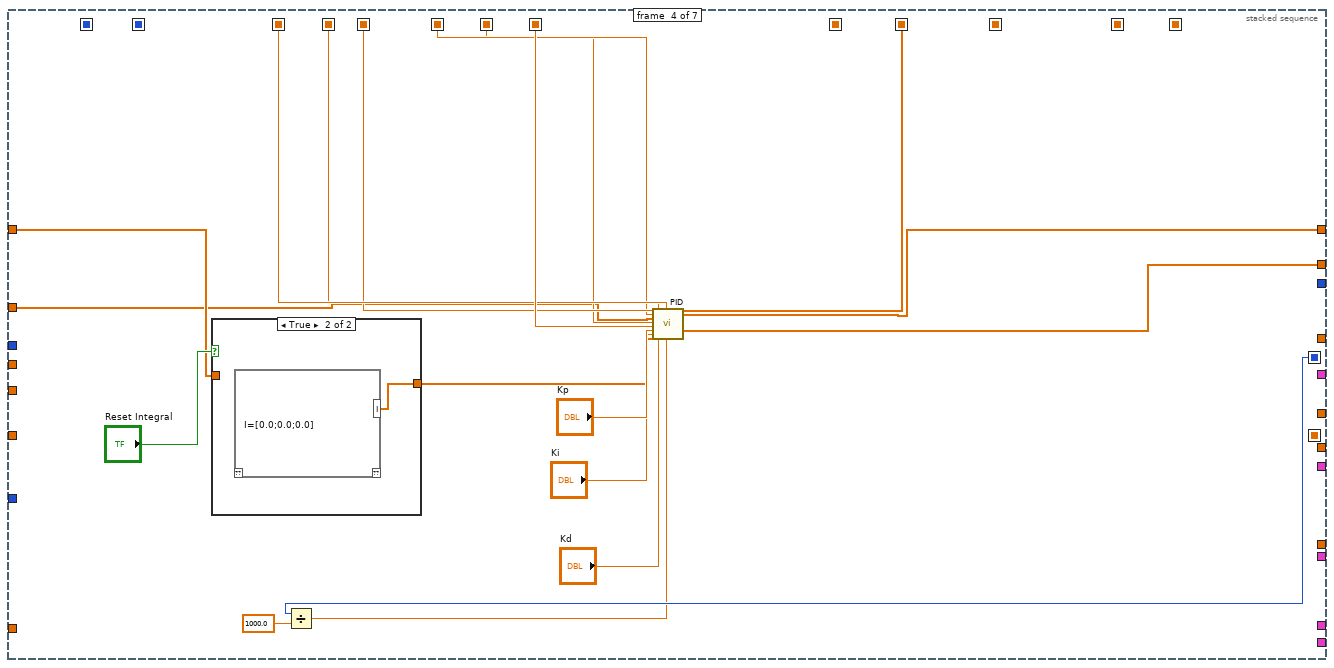
[diagram p6: hidden frame]
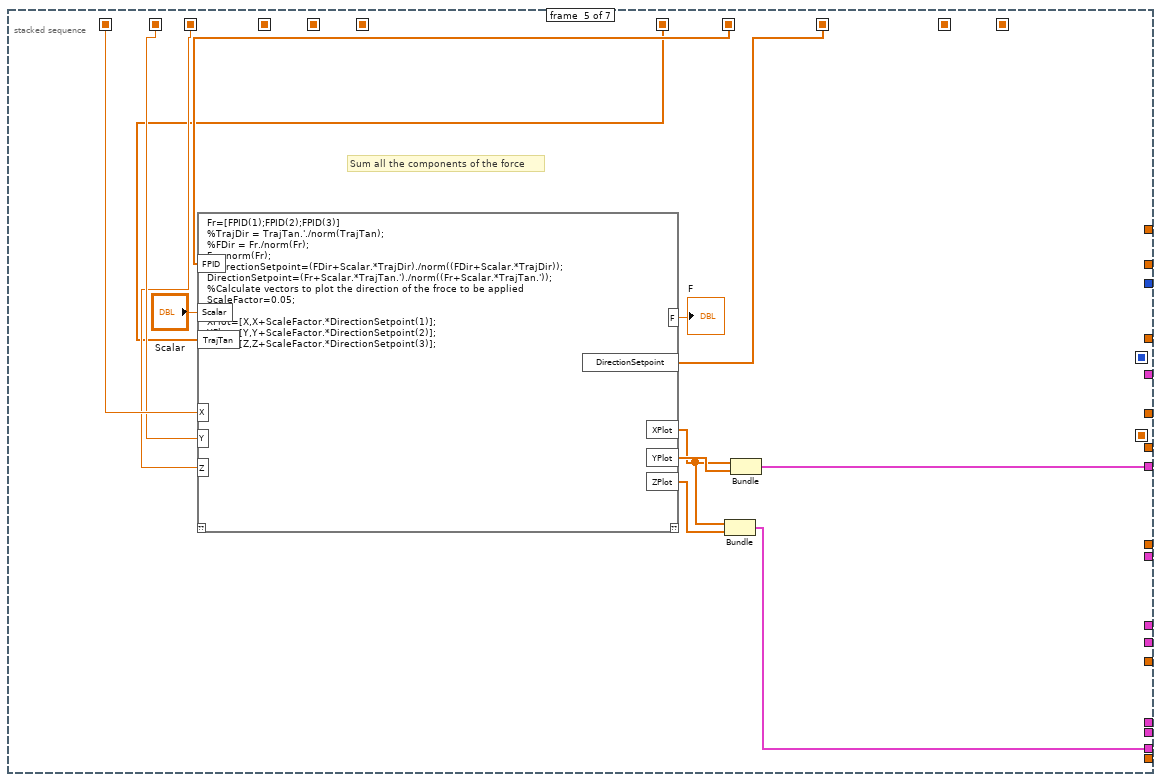
[diagram p8: hidden frame]
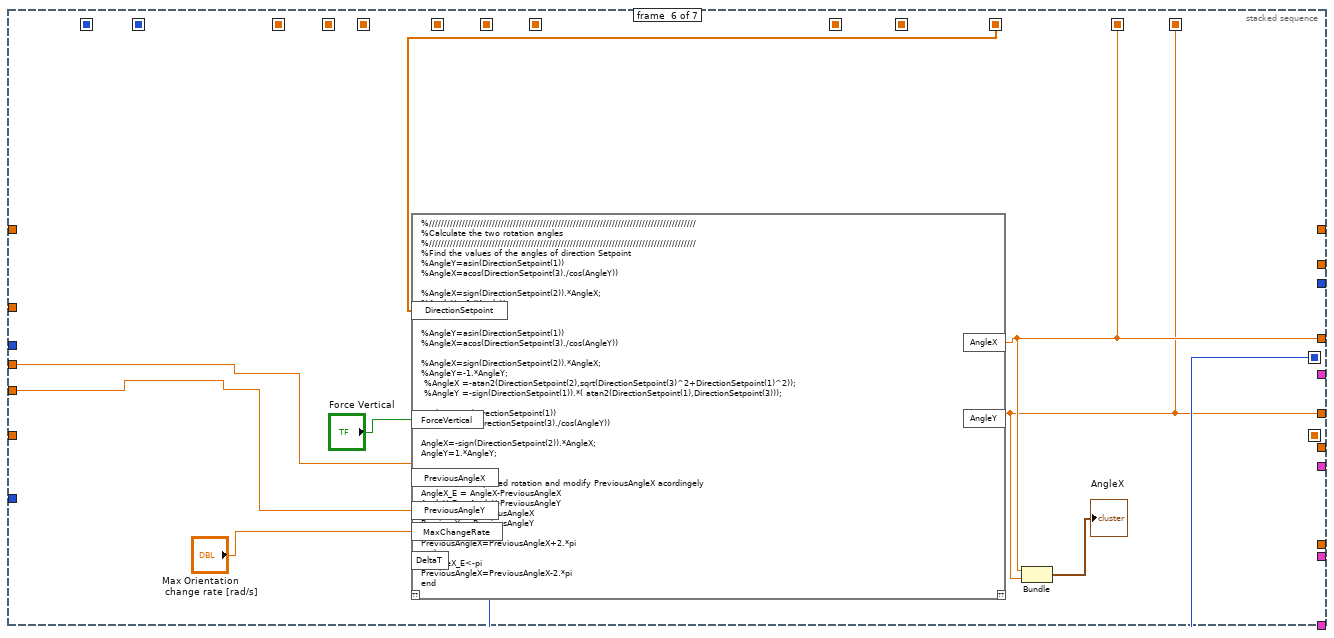
[diagram p9: hidden frame]
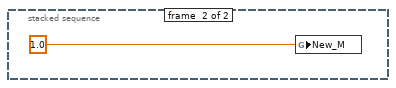
[diagram p11: hidden frame]
diagram:
  n1 = flat-sequence {
    tunnel: [w11] -> w6
    tunnel: [w11] -> w5
    tunnel: w6 -> [w14]
    tunnel: [w17] -> w4
    tunnel: [0.0] -> w3
    tunnel: [0.0] -> w2
    tunnel: [w13] -> w1
    tunnel: w4 -> [w59]
    tunnel: w3 -> [w57]
    tunnel: w2 -> [w58]
    tunnel: w1 -> [w60]
    frame #0 {
      n2 = Tick Count (ms)() -> (millisecond timer value=w11:u32)
    }
    frame #1 {
      n3 = mathscript code="I=[0.0;0.0;0.0]"() -> ("I"=w17:dbl[])  [unwired: 1 in, 1 out]
      n4 = Wait (ms)(milliseconds to wait=u32 2) -> ()  [unwired: 1 out]
      n5 = Subtract(x=w14, y=u32 1) -> (x-y=w13:u32)
    }
    frame #2 {
      n6 = property on="AngleX" class="WFChart (strict)"("History Data"=cluster{dbl, dbl}[] []) -> (error out=w56:errorcluster)  [unwired: 2 in, 1 out]
      n7 = property on="AngleX" class="WFChart (strict)"("History Data"=cluster{dbl, dbl}[] []) -> (error out=w52:errorcluster)  [unwired: 2 in, 1 out]
      n8 = property on="Error" class="WFChart (strict)"("History Data"=dbl[] []) -> (error out=w54:errorcluster)  [unwired: 2 in, 1 out]
      n9 = node-c288() -> (w62:T5)  [unwired: 4 in]
      n10 = timed-loop {
        timing: w62 -> [_]
        timing-out: [_] -> w61
        shift-right: [w93] -> _
        shift-left: w60 -> [w69]
        tunnel: w60 -> [w94]
        shift-right: [w78] -> _
        shift-left: w59 -> [w81]
        shift-right: [w79] -> _
        shift-left: w59 -> [w80]
        shift-right: [w73] -> _
        shift-left: w58 -> [w75]
        shift-right: [w72] -> _
        shift-left: w58 -> [w74]
        shift-right: [w71] -> _
        shift-left: w58 -> [w70]
        shift-right: [w65] -> _
        shift-left: w57 -> [w67]
        shift-right: [w64] -> _
        shift-left: w57 -> [w66]
        shift-right: [w63] -> _
        shift-left: w57 -> [w68]
        tunnel: w56 -> [_]
        tunnel: w54 -> [_]
        tunnel: w52 -> [_]
        stop <- "stop" stop-if-true
        n11 = node-c288() -> ()  [unwired: 1 in, 1 out]
        n12 = stacked-sequence {
          seq-local: [w98 _ _ _ _ _ _] -> [_ _ _ _ _ _ _]
          seq-local: [w99 _ _ _ _ _ _] -> [_ w104 _ _ _ _ _]
          seq-local: [w98 _ _ _ _ _ _] -> [_ _ _ w1200 _ w1472 w1936]
          seq-local: [_ w102 _ _ _ _ _] -> [_ _ w898 _ _ _ _]
          seq-local: [_ _ w893 _ _ _ _] -> [_ _ _ _ w1242 _ _]
          seq-local: [_ _ w892 _ _ _ _] -> [_ _ _ w1197 w1245 _ w1948]
          seq-local: [_ _ w891 _ _ _ _] -> [_ _ _ w1196 w1244 _ w1947]
          seq-local: [_ _ w890 _ _ _ _] -> [_ _ _ w1195 w1243 _ w1946]
          seq-local: [_ _ w889 _ _ _ _] -> [_ _ _ w1194 _ _ _]
          seq-local: [_ _ w888 _ _ _ _] -> [_ _ _ w1193 _ _ _]
          seq-local: [_ _ w887 _ _ _ _] -> [_ _ _ w1206 _ _ _]
          seq-local: [_ _ _ w1198 _ _ _] -> [_ _ _ _ w1246 _ _]
          seq-local: [_ _ _ _ w1249 _ _] -> [_ _ _ _ _ w1471 _]
          seq-local: [_ _ _ _ _ w1470 _] -> [_ _ _ _ _ _ w1939]
          seq-local: [_ _ _ _ _ w1469 _] -> [_ _ _ _ _ _ w1938]
          tunnel: w69 -> [w101 _ _ _ _ _ _]
          tunnel: w94 -> [w100 _ _ _ _ _ _]
          tunnel: [w97 _ _ _ _ _ _] -> w93
          tunnel: [_ _ w886 _ _ _ _] -> w87
          tunnel: [_ _ w885 _ _ _ _] -> w86
          tunnel: [_ _ w884 _ _ _ _] -> w85
          tunnel: [_ _ w883 _ _ _ _] -> w84
          tunnel: [_ _ w882 _ _ _ _] -> w83
          tunnel: [_ _ w881 _ _ _ _] -> w82
          tunnel: w81 -> [_ _ _ w1192 _ _ _]
          tunnel: w80 -> [_ _ _ w1191 _ _ _]
          tunnel: [_ _ _ w1190 _ _ _] -> w79
          tunnel: [_ _ _ w1189 _ _ _] -> w78
          tunnel: [_ _ _ _ w1248 _ _] -> w77
          tunnel: [_ _ _ _ w1247 _ _] -> w76
          tunnel: w75 -> [_ _ _ _ _ w1474 _]
          tunnel: w74 -> [_ _ _ _ _ w1473 _]
          tunnel: [_ _ _ _ _ w1470 _] -> w73
          tunnel: [_ _ _ _ _ w1469 _] -> w72
          tunnel: [_ _ _ _ _ _ w1943] -> w71
          tunnel: w70 -> [_ _ _ _ _ _ w1942]
          tunnel: w68 -> [_ _ _ _ _ _ w1928]
          tunnel: w67 -> [_ _ _ _ _ _ w1927]
          tunnel: w66 -> [_ _ _ _ _ _ w1926]
          tunnel: [_ _ _ _ _ _ w1925] -> w65
          tunnel: [_ _ _ _ _ _ w1924] -> w64
          tunnel: [_ _ _ _ _ _ w1923] -> w63
          frame #0 {
            n13 = Tick Count (ms)() -> (millisecond timer value=w97:u32)
            n14 = Subtract(x=w97, y=w101) -> (x-y=w98:u32)
            "Loop Duration [ms]" <- w98
            n15 = Subtract(x=w97, y=w100) -> (x-y=w99:u32)
          }
          frame #1 {
            # "This step generates the trajectory matrix"
            n16 = case shown="\"Stadium\", Default" "Radio Buttons" {
              tunnel: [w111 w619] -> w102
              tunnel: w104 -> [w113 _]
              tunnel: "XScale" -> [_ w615]
              tunnel: "Zoffset" -> [_ w616]
              tunnel: "Yoffset" -> [_ w618]
              tunnel: "Xoffset" -> [_ w617]
              tunnel: "Zscale" -> [_ w613]
              tunnel: "YScale" -> [_ w614]
              frame "Circle" {
                n17 = mathscript code="%////////////////////////////////////////////////////////////////////\n%Calculate the coordinates of the points on a circle that will define the\n%trajectory\n%////////////////////////////////////////////////////////////////////\nXCircle=[];\nYCircle=[];\nZCircle=[];\nVelocity=[];\nCircleRadius=0.03;\nAngleCircle=0;\ni=1;\nwhile true\n    XCircle(i,1)=CircleRadius.*cos(AngleCircle);\n    YCircle(i,1)=CircleRadius.*sin(AngleCircle);\n    ZCircle(i,1)=0;\n    Velocity(i,1)=100; %m/s\n    AngleCircle=AngleCircle+0.05;\n    i=i+1\n    if AngleCircle>2*pi\n        break\n    end\nend\n%////////////////////////////////////////////////////////////////////\n\n%/////////////////////////////////////////////////////////////////\n%Calculate rotation matrix\nAngleXTrajectory=0;\nif Traj_R\nAngleYTrajectory=0.1.*time./1000;\nelse\nAngleYTrajectory=0.*time./1000;\nend\nRotationMatrixX=[1 0 0;0 cos(-AngleXTrajectory) -sin(-AngleXTrajectory);0 sin(-AngleXTrajectory) cos(-AngleXTrajectory)];\nRotationMatrixY=[cos(-AngleYTrajectory) 0 sin(-AngleYTrajectory);0 1 0 ; -sin(-AngleYTrajectory) 0 cos(-AngleYTrajectory)];\nRotationMatrix=RotationMatrixX*RotationMatrixY;\n\n%Make the rotation\nTrajectoryTemp=[];\n\nfor k=1:length(XCircle)\n \n   TrajectoryTemp(:,k)=RotationMatrix*[XCircle(k);YCircle(k);ZCircle(k)];\nend\n%TrajectoryOut=TrajectoryOut';\nTrajectoryTemp=TrajectoryTemp'\n\nTrajectoryOut=[ TrajectoryTemp , Velocity]"("time"=w113, "Traj_R"="Traj_Rotate") -> ("TrajectoryOut"=w111:dbl[][])  [unwired: 1 in, 1 out]
              }
              frame "Stadium", Default {
                n18 = mathscript code="%////////////////////////////////////////////////////////////////////\n%Calculate the coordinates of the points on a circle that will define the\n%trajectory\n%////////////////////////////////////////////////////////////////////\nTraj=0.001*[-21,5.50000000000000,-18.3500000000000;-21,20.5000000000000,-18.5000000000000;-21,48,-18.5000000000000;-21,51,-19.1270000000000;-21,53.3000000000000,-20.6970000000000;-21,55.1840000000000,-23.8470000000000;-21,55.5000000000000,-28.5000000000000;-21,55.5000000000000,-48.5000000000000;-21,55.5000000000000,-68.5100000000000;-21,53.3000000000000,-73.8200000000000;-21,48,-76.0170000000000;-21,35.5960000000000,-76.0170000000000;-21,29.5900000000000,-76.0170000000000;-21,23.1920000000000,-76.0170000000000;-23.1970000000000,17.6970000000000,-76.0170000000000;-28.5000000000000,15.5000000000000,-76.0170000000000;-34.9500000000000,15.5000000000000,-76.0170000000000;-65.0500000000000,15.5000000000000,-76.0170000000000;-68.4300000000000,15.5000000000000,-76.0170000000000;-73.7300000000000,17.6900000000000,-76.0170000000000;-75.8600000000000,22.0340000000000,-76.0170000000000;-75.8600000000000,27.2700000000000,-76.0170000000000;-75.9300000000000,40.7900000000000,-76.0170000000000;-75.9300000000000,56.5400000000000,-76.0170000000000;-75.9300000000000,62.2900000000000,-76.0170000000000;-75.9300000000000,76.7600000000000,-76.0170000000000;-75.9300000000000,77.7600000000000,-75.5700000000000;-75.9300000000000,77.7600000000000,-74.5170000000000;-75.9300000000000,77.7600000000000,-70.7200000000000;-75.9300000000000,77.7600000000000,-60.2600000000000;-75.9300000000000,77.7600000000000,-21.3790000000000]\nTraj=[-0.0210000000000000,0.00550000000000000,-0.0183500000000000;-0.0210000000000000,0.0205000000000000,-0.0185000000000000;-0.0210000000000000,0.0480000000000000,-0.0185000000000000;-0.0210000000000000,0.0510000000000000,-0.0191270000000000;-0.0210000000000000,0.0533000000000000,-0.0206970000000000;-0.0210000000000000,0.0551840000000000,-0.0238470000000000;-0.0210000000000000,0.0555000000000000,-0.0285000000000000;-0.0210000000000000,0.0555000000000000,-0.0485000000000000;-0.0210000000000000,0.0555000000000000,-0.0685100000000000;-0.0210000000000000,0.0533000000000000,-0.0738200000000000;-0.0210000000000000,0.0480000000000000,-0.0760170000000000;-0.0210000000000000,0.0355960000000000,-0.0760170000000000;-0.0210000000000000,0.0295900000000000,-0.0760170000000000;-0.0210000000000000,0.0231920000000000,-0.0760170000000000;-0.0231970000000000,0.0176970000000000,-0.0760170000000000;-0.0285000000000000,0.0155000000000000,-0.0760170000000000;-0.0349500000000000,0.0155000000000000,-0.0760170000000000;-0.0650500000000000,0.0155000000000000,-0.0760170000000000;-0.0737300000000000,0.0176900000000000,-0.0760170000000000;-0.0758600000000000,0.0220340000000000,-0.0760170000000000;-0.0758600000000000,0.0272700000000000,-0.0760170000000000;-0.0759300000000000,0.0407900000000000,-0.0760170000000000;-0.0759300000000000,0.0565400000000000,-0.0760170000000000;-0.0759300000000000,0.0622900000000000,-0.0760170000000000;-0.0759300000000000,0.0767600000000000,-0.0760170000000000;-0.0759300000000000,0.0777600000000000,-0.0755700000000000;-0.0759300000000000,0.0777600000000000,-0.0745170000000000;-0.0759300000000000,0.0777600000000000,-0.0707200000000000;-0.0759300000000000,0.0777600000000000,-0.0602600000000000;-0.0759300000000000,0.0777600000000000,-0.0213790000000000]\n\n\n[m,n]=size(Traj)\n\nVelocity=zeros(m,1)+2000;\nxoffsetVect=zeros(m,1)+xoffset;\nyoffsetVect=zeros(m,1)+yoffset;\nzoffsetVect=zeros(m,1)+zoffset;\n\n\n%TrajectoryOut=[(Traj(:,1).*xscale) +xoffset,(Traj(:,2).*yscale) +yoffset,(Traj(:,3).*zscale) +zoffset, Velocity]\n\nTrajectoryOut=[xscale.*Traj(:,1)+xoffsetVect,-yscale.*Traj(:,3)+yoffsetVect,zscale.*Traj(:,2)+zoffsetVect, -Velocity]\n\n%TrajectoryOut=[xscale.*Traj(:,1)+xoffsetVect,-yscale.*Traj(:,3)+yoffsetVect,zscale.*Traj(:,2)+zoffsetVect, Velocity]\n\n\nFirstPoint=TrajectoryOut(1,:)\nTrajectoryOut=[TrajectoryOut]%;FirstPoint]\n%Test=TrajectoryOut(:,3)"("xscale"=w615, "yscale"=w614, "zscale"=w613, "zoffset"=w616, "yoffset"=w618, "xoffset"=w617) -> ("TrajectoryOut"=w619:dbl[][])  [unwired: 1 in, 1 out]
              }
            }
          }
          frame #2 {
            n19 = global read "Global 2.vi" "X"() -> (w892:dbl)
            n20 = global read "Global 2.vi" "Y"() -> (w891:dbl)
            n21 = global read "Global 2.vi" "Z"() -> (w890:dbl)
            n22 = call "TrajectoryControllerAhead.vi"("X"=w892, "Y"=w891, "Ahead"="Ahead", "Z"=w890, "Trajectory"=w898) -> ("error"=→"error" →"Error":cdb, "XHD"=w896:dbl[], "Xclosest"=w889:dbl, "Yclosest"=w888:dbl, "Zclosest"=w887:dbl, "ZHD"=w895:dbl[], "YHD"=w897:dbl[], "OptimumVelocity"=w893:dbl[])  [unwired: 3 in]
            n23 = mathscript code="XCircleBot=[];\nYCircleBot=[];\nZCircleBot = [];\nCircleRadius=0.002;\nAngleCircle=0;\ni=0\nwhile true\n     i=i+1\n    XCircleBot(i)=CircleRadius.*cos(AngleCircle);\n    YCircleBot(i)=CircleRadius.*sin(AngleCircle);\n    %ZCircleBot(i) = 0;\n    AngleCircle=AngleCircle+0.5;\n\n    if AngleCircle>2*pi\n        break\n    end\nend\nXCircleBotOut=XCircleBot+XPos;\nYCircleBotOut=YCircleBot+YPos;\nZCircleBotOut=YCircleBot+ZPos;\n\nXCircleClosestOut=XCircleBot+Xclosest;\nYCircleClosestOut=YCircleBot+Yclosest;\nZCircleClosestOut=YCircleBot+Zclosest;"("XPos"=w892, "YPos"=w891, "Xclosest"=w889, "Yclosest"=w888, "ZPos"=w890, "Zclosest"=w887) -> ("XCircleBotOut"=w902:dbl[], "YCircleBotOut"=w905:dbl[], "XCircleClosestOut"=w900:dbl[], "YCircleClosestOut"=w904:dbl[], "ZCircleClosestOut"=w901:dbl[], "ZCircleBotOut"=w903:dbl[])  [unwired: 1 in, 1 out]
            n24 = Bundle("XHD"=w896, "YHD"=w897) -> (w884:cluster{"XHD":dbl[], "YHD":dbl[]})  [unwired: 1 in]
            n25 = Bundle("XHD"=w896, "ZHD"=w895) -> (w883:cluster{"XHD":dbl[], "ZHD":dbl[]})  [unwired: 1 in]
            n26 = Bundle("XCircleClosestOut"=w900, "ZCircleClosestOut"=w901) -> (w881:T8)  [unwired: 1 in]
            n27 = Bundle("XCircleBotOut"=w902, "ZCircleBotOut"=w903) -> (w882:T9)  [unwired: 1 in]
            n28 = Bundle("XCircleClosestOut"=w900, "YCircleClosestOut"=w904) -> (w885:T10)  [unwired: 1 in]
            n29 = Bundle("XCircleBotOut"=w902, "YCircleBotOut"=w905) -> (w886:T11)  [unwired: 1 in]
          }
          frame #3 {
            n30 = case shown="True" "Reset Integral" {
              tunnel: w1192 -> [w1208 _]
              tunnel: [w1208 w1209] -> w1203
              frame False {
              }
              frame True {
                n31 = mathscript code="I=[0.0;0.0;0.0]"() -> ("I"=w1209:dbl[])  [unwired: 1 in, 1 out]
              }
            }
            n32 = Divide(x=w1200, y=1000.0) -> (x/y=w1199:dbl)
            n33 = call "PID.vi"("Z"=w1195, "Xclosest"=w1194, "ErrorIn"=w1191, "Yclosest"=w1193, "Zclosest"=w1206, "Kp"="Kp", "Ki"="Ki", "IntegralIn"=w1203, "Y"=w1196, "Kd"="Kd", "X"=w1197, "deltaT"=w1199) -> ("FPID"=w1198:dbl[], "IntegralOut"=w1189:dbl[], "ErrorOut"=w1190:dbl[])  [unwired: 13 in]
          }
          frame #4 {
            # "Sum all the components of the force"
            n34 = mathscript code="Fr=[FPID(1);FPID(2);FPID(3)]\n%TrajDir = TrajTan.'./norm(TrajTan);\n%FDir = Fr./norm(Fr);\nF = norm(Fr);\n%DirectionSetpoint=(FDir+Scalar.*TrajDir)./norm((FDir+Scalar.*TrajDir));\nDirectionSetpoint=(Fr+Scalar.*TrajTan.')./norm((Fr+Scalar.*TrajTan.'));\n%Calculate vectors to plot the direction of the froce to be applied\nScaleFactor=0.05;\n\nXPlot=[X,X+ScaleFactor.*DirectionSetpoint(1)];\nYPlot=[Y,Y+ScaleFactor.*DirectionSetpoint(2)];\nZPlot=[Z,Z+ScaleFactor.*DirectionSetpoint(3)];"("FPID"=w1246, "Y"=w1244, "Z"=w1243, "Scalar"="Scalar", "TrajTan"=w1242, "X"=w1245) -> ("DirectionSetpoint"=w1249:dbl[], "XPlot"=w1253:dbl[], "YPlot"=w1254:dbl[], "ZPlot"=w1252:dbl[], "F"=→"F":dbl)  [unwired: 1 in, 1 out]
            n35 = Bundle("XPlot"=w1253, "ZPlot"=w1252) -> (w1247:cluster{"XPlot":dbl[], "ZPlot":dbl[]})  [unwired: 1 in]
            n36 = Bundle("XPlot"=w1253, "YPlot"=w1254) -> (w1248:cluster{"XPlot":dbl[], "YPlot":dbl[]})  [unwired: 1 in]
          }
          frame #5 {
            n37 = mathscript code="%/////////////////////////////////////////////////////////////////////////////////////////\n%Calculate the two rotation angles\n%/////////////////////////////////////////////////////////////////////////////////////////\n%Find the values of the angles of direction Setpoint\n%AngleY=asin(DirectionSetpoint(1))\n%AngleX=acos(DirectionSetpoint(3)./cos(AngleY))\n\n%AngleX=sign(DirectionSetpoint(2)).*AngleX;\n%AngleY=-1.*AngleY;\n\n\n%AngleY=asin(DirectionSetpoint(1))\n%AngleX=acos(DirectionSetpoint(3)./cos(AngleY))\n\n%AngleX=sign(DirectionSetpoint(2)).*AngleX;\n%AngleY=-1.*AngleY;\n %AngleX =-atan2(DirectionSetpoint(2),sqrt(DirectionSetpoint(3)^2+DirectionSetpoint(1)^2));\n %AngleY =-sign(DirectionSetpoint(1)).*( atan2(DirectionSetpoint(1),DirectionSetpoint(3)));\n\nAngleY=asin(DirectionSetpoint(1))\nAngleX=acos(DirectionSetpoint(3)./cos(AngleY))\n\nAngleX=-sign(DirectionSetpoint(2)).*AngleX;\nAngleY=1.*AngleY;\n\n\n%Detect a completed rotation and modify PreviousAngleX acordingely\nAngleX_E = AngleX-PreviousAngleX\nAngleY_E = AngleY-PreviousAngleY\nPreviousX = PreviousAngleX\nPreviousY = PreviousAngleY\nif AngleX_E>pi\nPreviousAngleX=PreviousAngleX+2.*pi\nend\nif AngleX_E<-pi\nPreviousAngleX=PreviousAngleX-2.*pi\nend\n\n\n\nif AngleY_E>pi\nPreviousAngleX=PreviousAngleX+2.*pi\nend\nif AngleY_E<-pi\nPreviousAngleY=PreviousAngleY-2.*pi\nend\n\n\nVariationSpeedX=(AngleX-PreviousAngleX)./(DeltaT./1000)\nVariationSpeedY=(AngleY-PreviousAngleY)./(DeltaT./1000)\n\nif abs(VariationSpeedX)>MaxChangeRate\nAngleX=PreviousAngleX+MaxChangeRate.*(DeltaT./1000).*sign(VariationSpeedX)\nend\n\nif abs(VariationSpeedY)>MaxChangeRate\nAngleY=PreviousAngleY+MaxChangeRate.*(DeltaT./1000).*sign(VariationSpeedY)\nend\n\n%if abs(PreviousX-AngleX) > abs(AngleX+2*pi-PreviousX)\n%AngleX = AngleX + 2*pi\n%else\n%AngleX\n%end\n%if abs(PreviousY-AngleY) > abs(AngleY+2*pi-PreviousY)\n%AngleY = AngleY + 2*pi\n%else\n%AngleY\n%end\n\nif ForceVertical\nAngleX=0;\nAngleY=0;\nend"("DirectionSetpoint"=w1471, "ForceVertical"="Force Vertical", "PreviousAngleX"=w1474, "PreviousAngleY"=w1473, "MaxChangeRate"="Max Orientation\n change rate [rad/s]", "DeltaT"=w1472) -> ("AngleX"=w1470:cdb, "AngleY"=w1469:cdb)  [unwired: 1 in, 1 out]
            n38 = Bundle("AngleX"=w1470, "AngleY"=w1469) -> (→"AngleX":cluster{"AngleX":cdb, "AngleY":cdb})  [unwired: 1 in]
          }
          frame #6 {
            n39 = Multiply(x="RotationsPerSecond [Hz]", y=6.283185) -> (x*y=w1941:dbl)
            "RotationPerSecond[Hz]" <- w1941
            n40 = call "RotatingFieldCalculation_uvw.vi"("Time Step (ms)"=w1936, "Flux density magnitude (T)"="BMagnitude [T]", "Previous Field Angle (rad)"=w1942, "Omega (rad/s)"=w1941) -> ("Bv (T)"=w1944:sgl, "Bu (T)"=w1945:sgl, "New Field Angle (rad)"=w1943:sgl)  [unwired: 5 in]
            n41 = shared-variable "NI-IC-3173-01BA58CC\\EtherCAT Master\\Device\\Mod3\\TC7"() -> (→"Temperature":dbl)  [unwired: 1 in, 1 out]
            n42 = Divide(x=w1936, y=1000.0) -> (x/y=w1935:dbl)
            n43 = call "FieldPlaneRotation.vi"("Bv (T)"=w1944, "Bu (T)"=w1945, "AlfaY (rad)"=w1938, "AlfaX (rad)"=w1939) -> ("Bz (T)"=w1923:dbl, "By (T)"=w1924:dbl, "Bx (T)"=w1925:dbl)  [unwired: 5 in]
            n44 = Subtract(x=w1925, y=w1927) -> (x-y=w1932:dbl)
            n45 = Divide(x=w1932, y=w1935) -> (x/y=w1933:dbl)
            n46 = Subtract(x=w1923, y=w1928) -> (x-y=w1931:dbl)
            n47 = Divide(x=w1931, y=w1935) -> (x/y=w1929:dbl)
            n48 = Subtract(x=w1924, y=w1926) -> (x-y=w1930:dbl)
            n49 = Divide(x=w1930, y=w1935) -> (x/y=w1934:dbl)
            n50 = call "VoltageController.vi"("Y (m)"=w1947, "X (m)"=w1948, "dBzdt"=w1929, "Z (m)"=w1946, "dBxdt"=w1933, "Bx [T]"=w1925, "By [T]"=w1924, "Bz [T]"=w1923, "dBydt"=w1934) -> ("XN"=w1949:dbl, "XP"=w1954:dbl, "YN"=w1953:dbl, "YP"=w1952:dbl, "ZP"=w1950:dbl, "ZN"=w1951:dbl)  [unwired: 1 in]
            n51 = call "PowerSuppliesControlVoltageMode.vi"("Z-"=w1951, "OnOff"="Power On/Off", "Z+"=w1950, "Max Voltage (V)"=50.0, "Y-"=w1953, "Y+"=w1952, "X-"=w1949, "X+"=w1954) -> ("Saturating"=→"VoltageSaturating":bool)  [unwired: 3 in]
            "Power" <- "Power On/Off"
          }
        }
        n52 = Bundle(w87, w85, w86, w77) -> (w89:T12)  [unwired: 1 in]
        n53 = Bundle(w83, w84, w82, w76) -> (w91:T13)  [unwired: 1 in]
        n54 = Cluster To Array(cluster=w89) -> (array=→"XY View":cluster{"XPlot":dbl[], "YPlot":dbl[]}[])
        n55 = Cluster To Array(cluster=w91) -> (array=→"XZ View":cluster{"XPlot":dbl[], "ZPlot":dbl[]}[])
        n56 = node-c288() -> ()  [unwired: 1 in, 1 out]
      }
      n57 = node-c288(w61) -> ()  [unwired: 1 out]
    }
  }
  n58 = property on="coordinates" class="WFChart (strict)"("History Data"=cluster{dbl, dbl, dbl}[] []) -> (error out=w7:errorcluster)  [unwired: 2 in, 1 out]
  n59 = node-c288() -> (w10:T5)  [unwired: 4 in]
  n60 = timed-loop {
    timing: w10 -> [_]
    timing-out: [_] -> w9
    tunnel: w7 -> [_]
    shift-right: [w1968] -> _
    shift-left: w5 -> [w1969]
    shift-right: [w1967] -> _
    shift-left: _ -> [w1964]
    shift-right: [w1966] -> _
    shift-left: _ -> [w1963]
    shift-right: [w1965] -> _
    shift-left: _ -> [w1962]
    stop <- _ stop-if-true
    n61 = node-c288() -> ()  [unwired: 1 in, 1 out]
    n62 = stacked-sequence {
      tunnel: w1969 -> [w1982 _]
      tunnel: [w1981 _] -> w1968
      tunnel: [w1977 _] -> w1967
      tunnel: [w1976 _] -> w1966
      tunnel: [w1975 _] -> w1965
      tunnel: w1964 -> [w1974 _]
      tunnel: w1963 -> [w1973 _]
      tunnel: w1962 -> [w1972 _]
      frame #0 {
        w1998 = 296.0
        w2002 = sgl -0.00027  # Pixel size
        # "Machine Vision"
        # "Camera top"
        # "Machine Vision"
        # "Camera side"
        n63 = Tick Count (ms)() -> (millisecond timer value=w1981:u32)
        n64 = call "Vision Acquisition"() -> ("Image Out"=w2004:T3)  [unwired: 25 in, 2 out]
        n65 = call "Vision Acquisition2"() -> ("Image Out"=w2015:T3)  [unwired: 25 in, 2 out]
        n66 = Subtract(x=w1981, y=w1982) -> (x-y=→"camera rate":u32)
        n67 = call "IMAQ Count Objects 2"("Settings"="Settings 3", "Image"=w2004) -> ("Image Out"=→"Image 3":T3, "Objects"=w2008:T14)  [unwired: 5 in, 3 out]
        n68 = call "IMAQ Count Objects 2"("Settings"="Settings 4", "Search Rect (entire image)"="Search Rect (entire image)", "Image"=w2015) -> ("Image Out"=→"Image 4":T3, "Objects"=w2014:T14)  [unwired: 4 in, 3 out]
        n69 = Array To Cluster(array=w2008) -> (cluster=w2007:T15)
        n70 = Array To Cluster(array=w2014) -> (cluster=w2013:T15)
        n71 = Unbundle(w2007) -> ("Objects[0]"=w2006:T16)  [unwired: 8 out]
        n72 = Unbundle(w2013) -> ("Objects[0]"=w2012:T16)  [unwired: 8 out]
        n73 = Unbundle(w2006) -> ("Object Center"=w2005:cluster{"X":sgl, "Y":sgl})  [unwired: 5 out]
        n74 = Unbundle(w2012) -> ("Object Center"=w2011:cluster{"X":sgl, "Y":sgl})  [unwired: 5 out]
        n75 = Unbundle(w2005) -> ("X"=w1996:sgl, "Y"=w1993:sgl)
        n76 = Unbundle(w2011) -> ("X"=w1995:sgl, "Y"=w1994:sgl)
        n77 = Subtract(x=w1995, y=w1998) -> (x-y=w2001:dbl)
        n78 = Subtract(x=w1993, y=w1998) -> (x-y=w1999:dbl)
        n79 = Subtract(x=w1994, y=w1998) -> (x-y=w2000:dbl)
        n80 = Multiply(x=w2001, y=sgl 0.00027) -> (x*y=w1989:dbl)
        n81 = Multiply(x=sgl -0.00027 ("y"), y=w2000) -> (x*y=w1988:dbl)
        n82 = Multiply(x=w1996, y=w2002) -> ()  [unwired: 1 out]
        n83 = Multiply(x=w2002, y=w1999) -> (x*y=w1987:dbl)
        n84 = mathscript code="FOVX=0.6*1.6; %field of view on x axis\nFOVY=0.6*1.6; %field of view on y axis\nFOVZ=0.6*1.6; %field of view on z axis\n\nNbPixelsX=592;\nNbPixelsY=592;\nNbPixelsZ=592;\n\nCOX=0.26*1.2; %camera offset fromc enter\nCOY=0.26*1.2; %camera offset fromc enter\nCOZ=0.26*1.2; %camera offset fromc enter\n\n\ntanAngleX=((Xin-(NbPixelsX/2))/NbPixelsX)*tan(FOVX/2);\ntanAngleY=(((NbPixelsY-Yin)-(NbPixelsY/2))/NbPixelsY)*tan(FOVY/2);\ntanAngleZ=(((NbPixelsZ-Zin)-(NbPixelsZ/2))/NbPixelsZ)*tan(FOVZ/2);\n\nX=(COX*tanAngleX-tanAngleX*COZ*tanAngleZ)./(1-tanAngleX*tanAngleY)\nZ=(COZ-X)*tanAngleZ\nY=(COY-Z)*tanAngleY\n\nX = round(X*10000)/10000\nY = round(Y*10000)/10000\nZ = round(Z*10000)/10000\n\nerror = sqrt((X-X_last_in).^2+(Y-Y_last_in).^2+(Z-Z_last_in).^2);\nif error > 0.09\nindicat = true\nX = X_last_in\nY=Y_last_in\nZ= Z_last_in\nelse\nindicat = false\nend\n\nX_last_out = X\nY_last_out = Y\nZ_last_out = Z"("Xin"=w1995, "Yin"=w1994, "Zin"=w1993, "X_last_in"=w1974, "Y_last_in"=w1973, "Z_last_in"=w1972) -> ("X"=w1980:dbl, "Y"=w1991:dbl, "Z"=w1990:dbl, "indicat"=→"Error_detection":bool, "error"=→"Detection_Error":dbl, "X_last_out"=w1977:dbl, "Y_last_out"=w1976:dbl, "Z_last_out"=w1975:dbl)  [unwired: 1 in, 1 out]
        n85 = case shown="False" "Vision compensation" {
          tunnel: [w2020 w2023] -> w1970
          tunnel: w1980 -> [_ w2023]
          tunnel: [w2019 w2022] -> w1985
          tunnel: w1991 -> [_ w2022]
          tunnel: [w2018 w2021] -> w1984
          tunnel: w1990 -> [_ w2021]
          tunnel: w1989 -> [w2020 _]
          tunnel: w1988 -> [w2019 _]
          tunnel: w1987 -> [w2018 _]
          frame False {
          }
          frame True {
          }
        }
        "X" <- w1970
        "Y" <- w1985
        "Z" <- w1984
        n86 = global write "Global 2.vi" "Y"(w1985) -> ()
        n87 = global write "Global 2.vi" "Z"(w1984) -> ()
        n88 = global write "Global 2.vi" "X"(w1970) -> ()
        n89 = Bundle("X"=w1970, "Y"=w1985, "Z"=w1984) -> (→"coordinates":cluster{"X":dbl, "Y":dbl, "Z":dbl})  [unwired: 1 in]
        "Vision compensation active" <- "Vision compensation"
      }
      frame #1 {
        n90 = global write "Global 2.vi" "New_M"(1.0 ("New_M")) -> ()
      }
    }
    n91 = node-c288() -> ()  [unwired: 1 in, 1 out]
  }
  n92 = node-c288(w9) -> ()  [unwired: 1 out]
